vi "Send Image.vi"(8 "error in (no error)":errorcluster, 10 "notifier":refnum<notifier>, 11 "Camera Address":string) -> (0 "error out":errorcluster, 2 "notifier out":refnum<notifier>)   [LabVIEW 2015]
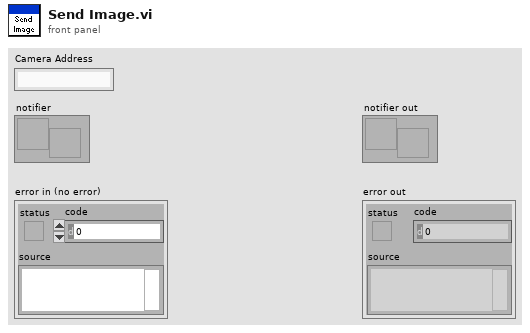
[diagram p1: front panel]
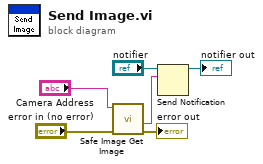
[diagram p0: block diagram]
diagram:
  n1 = call <vilib>:"Safe Image Get Image.vi"("error in"="error in (no error)", "Session In"="Camera Address") -> ("error out"=→"error out":errorcluster, "Image Data String"=w4:string)  [unwired: 6 in, 2 out]
  n2 = Send Notification(notification=w4, notifier="notifier") -> (notifier out=→"notifier out":refnum<notifier>)  [unwired: 1 in, 1 out]
